vi "VMA.vi"(0 "System no.":i32=1 min=1 max=4 step=1, 2 "Axes to set":string[](array[string]), 3 "Upper PZT limit (V)":dbl[](array[numeric]) format="%.6f", 4 "No.of digits":i16=4, 5 "error in":errorcluster) -> (14 "Controller error":bool, 19 "error out":errorcluster)   [LabVIEW 2020]
doc: "Sets upper voltage limit for all PZTs affected by specified axes. No. of digits is the number of digits after the decimal point in the limit value(s) that will be sent. Controller error is TRUE if selected system reports an error code which is not 0.\n\nE-516: The VMA command saves the parameters in RAM only. To save the currently valid parameters to flash ROM, where they become the power-on defaults, you must run WPA.vi. Parameter changes not saved with WPA will be lost when the controller is powered off.\n\nE-517, E-518: Axes to set are piezo channel numbers.The VMA command saves the parameters in RAM only. To save the currently valid parameters to flash ROM, where they become the power-on defaults, you must run WPA.vi. Parameter changes not saved with WPA will be lost when the controller is powered off.\n\nE-710: Axes to set are piezo numbers. Command is available in command level 1 only (see CCL.vi and CCL?.vi)\n\nE-761: Axes to set are piezo channel numbers, which can be 1 to 4. Use \"WPA.vi\" to save currently valid parameters. When booting the E-761, the value is replaced by the \"Max. Voltage of Amplifier\" parameter, but can be restored with RPA."
panel:
  # "Sets the upper PZT voltage limit and checks for error."
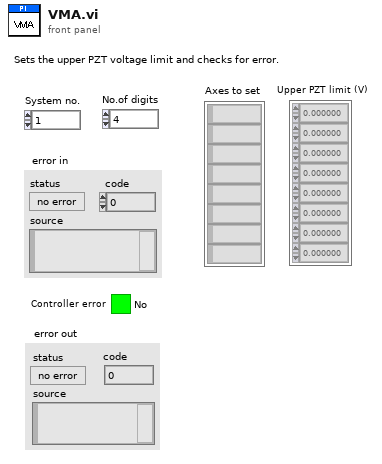
[diagram p1: front panel]
types:
  T1 = enum16{"Disable error check", "Force error check", "Use global settings"}
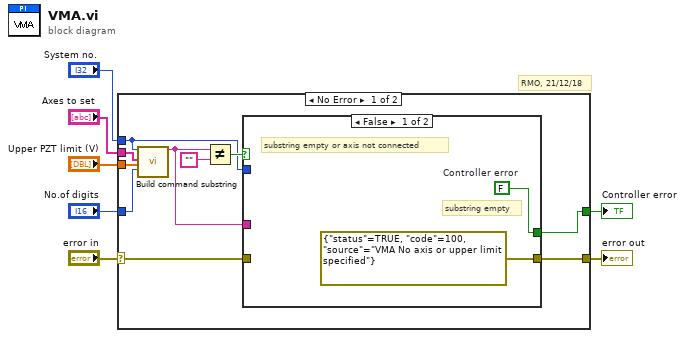
[diagram p0: block diagram]
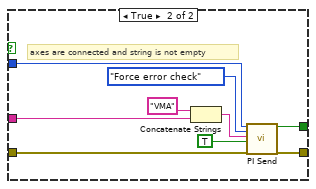
[diagram p2: hidden frame]
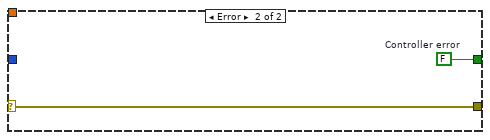
[diagram p3: hidden frame]
diagram:
  # "RMO, 21/12/18"
  n1 = case shown="No Error" "error in" {
    selector: "error in" -> [w8 w29]
    tunnel: [w17 w29] -> w7
    tunnel: "Upper PZT limit (V)" -> [w14 _]
    tunnel: "No.of digits" -> [w13 _]
    tunnel: "System no." -> [w10 _]
    tunnel: "Axes to set" -> [w12 _]
    tunnel: [w9 w30] -> w2
    frame No Error {
      n2 = call "Build command substring.vi"("System no."=w10, "Affected axes"=w12, "Parameters"=w14, "No. of digits"=w13) -> ("Command substring"=w15:string)  [unwired: 3 in, 12 out]
      n3 = Not Equal?(x=w15, y="") -> (x != y?=w11:bool)
      n4 = case shown="False" w11 {
        tunnel: w15 -> [_ w27]
        tunnel: [errorcluster {"status"=TRUE, "code"=100, "source"="VMA No axis or upper limit specified"} ("error out") w21] -> w17
        tunnel: w8 -> [_ w24]
        tunnel: w10 -> [_ w23]
        tunnel: [w18 w20] -> w9
        frame False {
          w18 = FALSE  # Controller error
          # "substring empty"
          # "substring empty or axis not connected"
        }
        frame True {
          # "axes are connected and string is not empty"
          n5 = Concatenate Strings("VMA", w27) -> (w25:string)
          n6 = call "PI Send.vi"("System no."=w23, "Error check settings"=T1."Force error check", "String to send"=w25, "Attach termination char.?"=TRUE ("Attach Linefeed?"), "error in"=w24) -> ("Controller error"=w20:bool, "error out"=w21:errorcluster)  [unwired: 1 in, 12 out]
        }
      }
    }
    frame Error {
      w30 = FALSE  # Controller error
    }
  }
  "error out" <- w7
  "Controller error" <- w2
